vi "wf_array_adjust_t0.vi"(8 "error in":errorcluster, 10 "scope in":waveform(dbl)[](array[waveform]), 11 "position":dbl format="%#_13g") -> (0 "error out":errorcluster, 2 "scope out":waveform(dbl)[](array[waveform]))   [LabVIEW 2017, in "tools.lvlib"]
uses:
  tools.lvlib
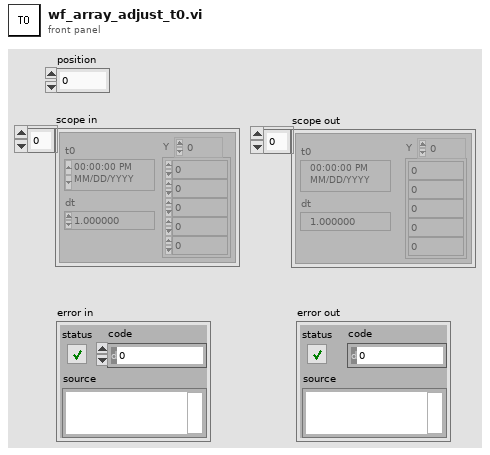
[diagram p1: front panel]
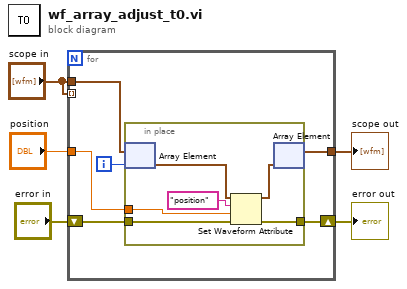
[diagram p0: block diagram]
diagram:
  n1 = for {
    tunnel: "scope in" -> [w11]
    tunnel: [w9] -> w4
    tunnel: "position" -> [w8]
    shift-right: [w6] -> w2
    shift-left: "error in" -> [w7]
    tunnel: "scope in" -> [_] mode=indexing
    i -> [w10]
    n2 = in-place {
      in-place-border: w8 -> [w14]
      in-place-border: w7 -> [w13]
      in-place-border: [w12] -> w6
      n3 = in-place-array #1(w11, w10) -> (w17:waveform(dbl))
      n4 = Set Waveform Attribute(4:w13, 5:w14, 6:"position" ("name"), 7:w17) -> (0:w12:errorcluster, 3:w16:waveform(dbl))  [unwired: 1 out]
      n5 = in-place-array #1(w16) -> (w9:waveform(dbl)[])  [unwired: 1 out]
    }
  }
  "scope out" <- w4
  "error out" <- w2
